vi "Add Subscriber.vi"(8 "error in (no error)":errorcluster, 10 "New FIFO Instance Config":T1, 11 "CIFChannels in":refnum<class "CIFChannels.lvclass">) -> (0 "error out":errorcluster, 2 "New Publisher":string, 3 "CIFChannels out":refnum<class "CIFChannels.lvclass">)   [LabVIEW 2021, in "CIFChannels.lvclass"]
uses:
  CIFChannels.lvclass
  CIFChannels.lvclass/CIFChannels.ctl
  ChannelCommon/ChannelCommon.lvlib
  ChannelCommon/typedef/Errors.ctl
  ChannelCommon/typedef/New FIFO Instance Configuration.ctl
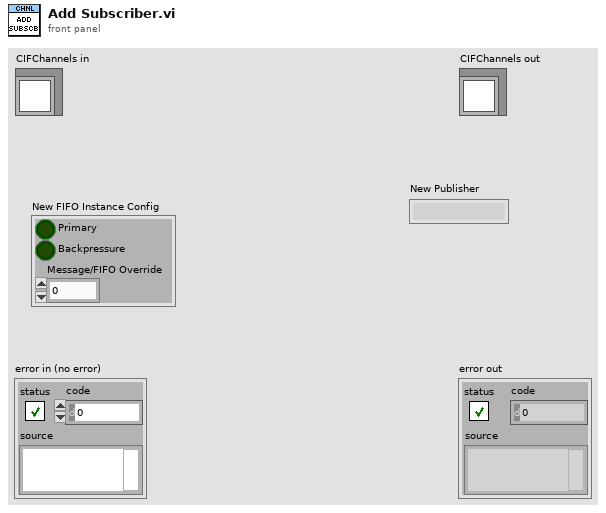
[diagram p1: front panel]
types:
  T1 = typedef "ChannelCommon.lvlib/New FIFO Instance Configuration.ctl" = cluster{"Primary":bool, "Backpressure":bool, "Message/FIFO Override":u32}
  T2 = typedef "ChannelCommon.lvlib/Errors.ctl" = enum16{"gRPC Server Not Found", "Duplicate Channel", "Missing Channel", "Incorrect Type", "Flatten Error", "Unflatten Data", "Channel Length", "Plugin Connection", "gRPC Server Connection", "FIFO Unflatten", "Required Override", "Remove Not Found", "Not Supported"}
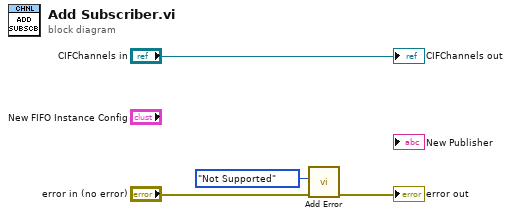
[diagram p0: block diagram]
diagram:
  n1 = call "Add Error.vi"("error in (no error)"="error in (no error)", "Error"=Errors."Not Supported") -> ("error out"=→"error out":errorcluster)  [unwired: 9 in]
  "CIFChannels out" <- "CIFChannels in"
